vi "re_LuaVIEW Poll Print Buffer_srv.vi"(0 "timeout":u32, 5 "read all?":bool, 7 "certificate":string, 9 "read index in":i32, 11 "task identifier":string) -> (4 "text":string, 6 "text gap?":bool, 10 "read index out":i32, 15 "error out":errorcluster)   [LabVIEW 2012]
doc: "Remote-calling wrapper around the \"Poll Print Buffer\" advanced API VI. Does retries until timeout to reduce network traffic."
uses:
  clientsrv/typedefs/t_ClientSrv Access Levels.ctl
  typedefs/t_LuaVIEW Task List Methods.ctl
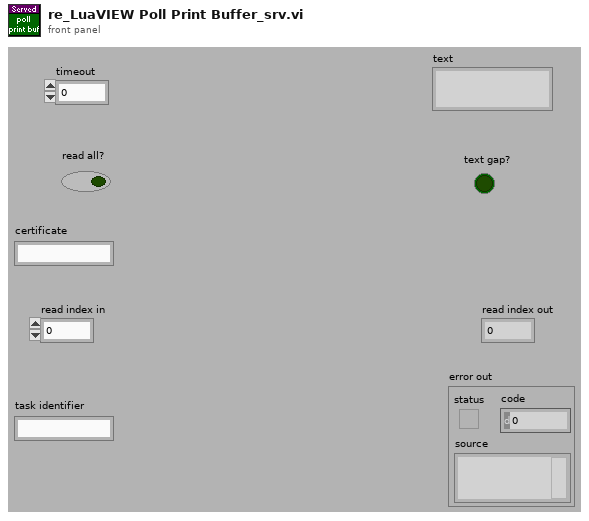
[diagram p1: front panel]
types:
  T1 = typedef "t_ClientSrv Access Levels.ctl" = enum16{"observer", "operator", "local"}
  T2 = typedef "t_LuaVIEW Task List Methods.ctl" = enum16{"clear list", "add", "test", "remove", "get ref", "get task info", "get list", "get script info", "ongoing?", "resume", "pause", "stop", "confirm", "message"}
  T3 = typedef "LuaVIEW Task Info.ctl" = cluster{"main script":string, "identifier":string, "class":string, "description":string, "mode":T4, "handler":string, "LuaVIEW reference":T5, "scripts":i32, "hide":bool, "active":bool, "error msg":string, "defer":bool, "launch":enum16{"asynchronous", "manual", "synchronous"}, "main path valid":bool, "start time":dbl, "swap time":dbl, "task VI":refnum<vi>, "prefsys":enum32{"invalid execution system", "user interface", "standard", "instrument i/o", "data acquisition", "other 1", "other 2", "same as caller"}, "priority":enum32{"invalid priority", "background priority", "normal priority", "above normal priority", "high priority", "time critical priority", "subroutine"}, "signal flags":u32, "allow mask":u32, "handle mask":u32, "disallow manual":bool}
  T4 = typedef "t_LuaVIEW Task Modes.ctl" = enum16{"initializing", "running", "executing", "paused", "error", "swapping"}
  T5 = typedef "t_LuaVIEW Reference.ctl" = refnum<k1>
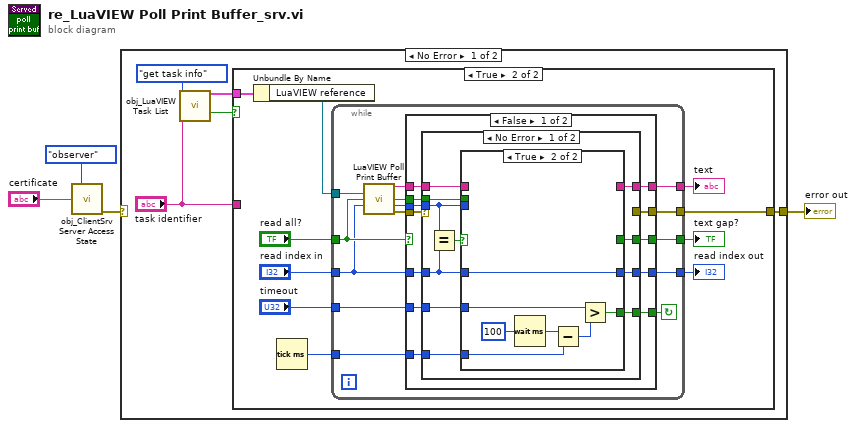
[diagram p0: block diagram]
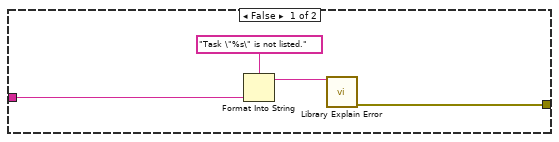
[diagram p2: hidden frame]
diagram:
  n1 = call "obj_ClientSrv Server Access State.vi"("access level"=t_ClientSrv_Access_Levels."observer", "certificate in"="certificate") -> ("error out"=w2:errorcluster)  [unwired: 11 in, 2 out]
  n2 = case shown="No Error" w2 {
    selector: w2 -> [_ w77]
    tunnel: [w5 w77] -> w1
    frame No Error {
      n3 = call "obj_LuaVIEW Task List.vi"("method"=t_LuaVIEW_Task_List_Methods."get task info", "task identifier"="task identifier") -> ("task info"=w8:T3, "set/ongoing"=w7:bool)  [unwired: 8 in, 4 out]
      n4 = case shown="True" w7 {
        tunnel: w8 -> [_ w23]
        tunnel: "task identifier" -> [w13 _]
        tunnel: [w10 w21] -> w5
        frame False {
          n5 = Format Into String(format string="Task \"%s\" is not listed.", w13) -> (resulting string=w11:string)  [unwired: 2 in, 1 out]
          n6 = call "Library Explain Error.vi"("explanation prefix (none)"=w11) -> ("explained error"=w10:errorcluster)  [unwired: 14 in]
        }
        frame True {
          n7 = Unbundle By Name(w23) -> ("LuaVIEW reference"=w22:T5)
          n8 = Tick Count (ms)() -> (millisecond timer value=w15:u32)
          n9 = while {
            tunnel: w22 -> [w37]
            tunnel: [w32] -> w21
            tunnel: "read all?" -> [w36]
            tunnel: "read index in" -> [w27]
            tunnel: [w30] -> w18
            tunnel: [w35] -> w17
            tunnel: [w33] -> w16
            tunnel: w15 -> [w26]
            tunnel: "timeout" -> [w25]
            stop <- w24 continue-if-true
            n10 = call "LuaVIEW Poll Print Buffer.vi"("LuaVIEW reference in"=w37, "read all?"=w36, "read index in"=w27) -> ("text"=w34:string, "text gap?"=w28:bool, "read index out"=w29:i32, "error out"=w31:errorcluster)  [unwired: 8 in, 1 out]
            n11 = case shown="False" w36 {
              tunnel: [w45 w73] -> w35
              tunnel: w34 -> [w48 w76]
              tunnel: [w47 w76] -> w33
              tunnel: w31 -> [w49 w75]
              tunnel: [w46 w75] -> w32
              tunnel: [w43 w74] -> w30
              tunnel: w29 -> [w42 w74]
              tunnel: w28 -> [w44 w73]
              tunnel: w27 -> [w41 _]
              tunnel: w26 -> [w40 _]
              tunnel: w25 -> [w39 _]
              tunnel: [w38 _] -> w24
              frame False {
                n12 = case shown="No Error" w49 {
                  selector: w49 -> [_ w72]
                  tunnel: w48 -> [w59 _]
                  tunnel: [w58 _] -> w47
                  tunnel: [_ w72] -> w46
                  tunnel: [w57 _] -> w45
                  tunnel: w44 -> [w55 _]
                  tunnel: [w56 w71] -> w43
                  tunnel: w42 -> [w54 _]
                  tunnel: w41 -> [w50 w71]
                  tunnel: w40 -> [w53 _]
                  tunnel: w39 -> [w52 _]
                  tunnel: [w51 _] -> w38
                  frame No Error {
                    n13 = Equal?(x=w54, y=w50) -> (x = y?=w60:bool)
                    n14 = case shown="True" w60 {
                      tunnel: [w63 _] -> w58
                      tunnel: w59 -> [w63 _]
                      tunnel: [w62 _] -> w57
                      tunnel: [w61 w64] -> w56
                      tunnel: w55 -> [w62 _]
                      tunnel: w54 -> [w61 _]
                      tunnel: w53 -> [_ w68]
                      tunnel: w52 -> [_ w67]
                      tunnel: [_ w65] -> w51
                      tunnel: w50 -> [_ w64]
                      frame False {
                      }
                      frame True {
                        n15 = Wait (ms)(milliseconds to wait=u32 100) -> (millisecond timer value=w69:u32)
                        n16 = Subtract(x=w69, y=w68) -> (x-y=w66:u32)
                        n17 = Greater?(x=w67, y=w66) -> (0:w65:bool)
                      }
                    }
                  }
                  frame Error {
                  }
                }
              }
              frame True {
              }
            }
          }
          "read index out" <- w18
          "text gap?" <- w17
          "text" <- w16
        }
      }
    }
    frame Error {
    }
  }
  "error out" <- w1
